vi "Launch Command Loop.vi"(7 "VI Refnum":refnum<vi>, 8 "error in":errorcluster, 10 "Queue Refs":variant, 11 "Device Reference in":T1=18446744073709551615 format="%.0x") -> (0 "error out":errorcluster)   [LabVIEW 2026, in "Runtime Configuration Support Inline Async Example Custom Device Engine.lvlib"]
uses:
  <vilib>/NI VeriStand/Custom Device API/Custom Device Item Ref.ctl
  Runtime Configuration Support Inline Async Example Custom Device Engine.lvlib
  <vilib>/NI VeriStand/Custom Device API/Custom Device API.lvlib
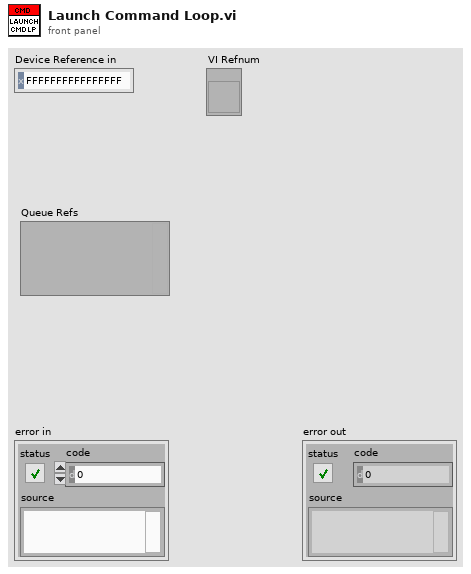
[diagram p1: front panel]
types:
  T1 = typedef "Custom Device API.lvlib/Custom Device Item Ref.ctl" = u64
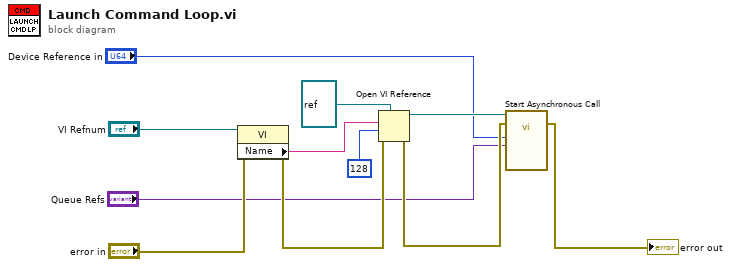
[diagram p0: block diagram]
diagram:
  n1 = property class="VI"(reference="VI Refnum", error in="error in") -> (error out=w11:errorcluster, "Name"=w6:string)  [unwired: 1 out]
  n2 = Open VI Reference(type specifier VI Refnum (for type only)=refnum<vi> refnum, vi path=w6, options=128, error in (no error)=w11) -> (vi reference=w3:refnum<vi>, error out=w9:errorcluster)  [unwired: 2 out]
  n3 = call-by-ref "Start Asynchronous Call"(reference=w3, error in=w9, "Queue Refs"="Queue Refs", "Device Reference in"="Device Reference in") -> (error out=→"error out":errorcluster)  [unwired: 10 in, 1 out]
